vi "SERIAL_StoreBuffer.vi"(8 "error in (no error)":errorcluster, 9 "Access Type":enum16{"set", "get", "delete"}(ring), 10 "navX Data":u8[](array[numeric]), 11 "SerialPortRef":T1) -> (0 "error out":errorcluster, 2 "navX Data":u8[](array[numeric]), 3 "SerialPortRef":T1)   [LabVIEW 2014, in "navX-MXP IMU.lvlib"]
uses:
  navX-MXP IMU.lvlib
  <vilib>/Rock Robotics/WPI/SerialPort/WPI_SerialPortRef.ctl
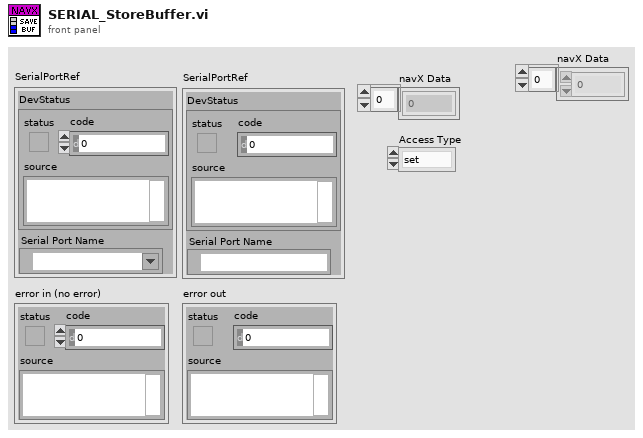
[diagram p1: front panel]
types:
  T1 = typedef "WPI_SerialPortRef.ctl" = cluster{"DevStatus":errorcluster, "Serial Port Name":refnum<visa-resource-name>}
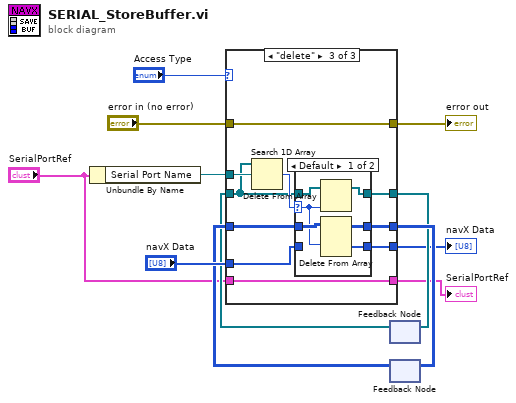
[diagram p0: block diagram]
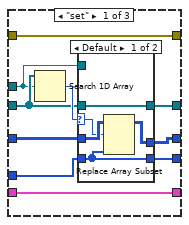
[diagram p2: hidden frame]
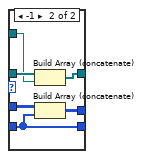
[diagram p3: hidden frame]
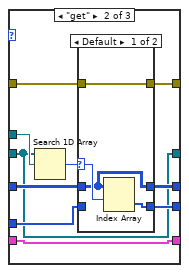
[diagram p4: hidden frame]
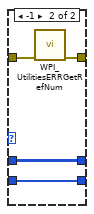
[diagram p5: hidden frame]
diagram:
  n1 = Unbundle By Name("SerialPortRef") -> ("Serial Port Name"=w8:refnum<visa-resource-name>)
  n2 = feedback #1() -> (w7:refnum<visa-resource-name>[])  [unwired: 1 in]
  n3 = feedback #2() -> (w9:u8[][])  [unwired: 1 in]
  n4 = case shown="\"delete\"" "Access Type" {
    tunnel: "navX Data" -> [w21 w36 w53]
    tunnel: [w20 w39 w55] -> w10
    tunnel: w9 -> [w19 w38 w54]
    tunnel: w8 -> [w15 w43 w61]
    tunnel: w7 -> [w17 w35 w58]
    tunnel: [w18 w35 w59] -> w6
    tunnel: [w13 w34 w57] -> w5
    tunnel: "SerialPortRef" -> [w13 w34 w57]
    tunnel: [w16 w40 w56] -> w3
    tunnel: "error in (no error)" -> [w16 w41 w56]
    tunnel: [w14 w37 w52] -> w1
    frame "set" {
      n5 = Search 1D Array(1D array=w17, element=w15) -> (index of element=w22:i32)  [unwired: 1 in]
      n6 = case shown="Default" w22 {
        selector: w22 -> [w23 _]
        tunnel: w21 -> [w24 w28]
        tunnel: [w27 w29] -> w20
        tunnel: w19 -> [w26 w30]
        tunnel: [w25 w31] -> w18
        tunnel: w17 -> [w25 w33]
        tunnel: w15 -> [_ w32]
        tunnel: [w24 w28] -> w14
        frame Default {
          n7 = Replace Array Subset(array=w26, new element=w24, index (row)=w23) -> (w27:u8[][])  [unwired: 1 in]
        }
        frame -1 {
          n8 = Build Array (concatenate)(w33, w32) -> (w31:refnum<visa-resource-name>[])
          n9 = Build Array (concatenate)(w30, w28) -> (w29:u8[][])
        }
      }
    }
    frame "get" {
      n10 = Search 1D Array(1D array=w35, element=w43) -> (index of element=w42:i32)  [unwired: 1 in]
      n11 = case shown="Default" w42 {
        selector: w42 -> [w47 _]
        tunnel: w41 -> [w45 w51]
        tunnel: [w45 w50] -> w40
        tunnel: [w44 w49] -> w39
        tunnel: w38 -> [w44 w49]
        tunnel: [w46 w48] -> w37
        tunnel: w36 -> [_ w48]
        frame Default {
          n12 = Index Array(array=w44, index (row)=w47) -> (element=w46:u8[])  [unwired: 1 in]
        }
        frame -1 {
          n13 = call <vilib>:"WPI_UtilitiesERRGetRefNum.vi"("error in (no error)"=w51) -> ("ERRGetRefNum"=w50:errorcluster)  [unwired: 10 out]
        }
      }
    }
    frame "delete" {
      n14 = Search 1D Array(1D array=w58, element=w61) -> (index of element=w60:i32)  [unwired: 1 in]
      n15 = case shown="Default" w60 {
        selector: w60 -> [w65 _]
        tunnel: [w62 w70] -> w59
        tunnel: w58 -> [w67 w70]
        tunnel: [w64 w69] -> w55
        tunnel: w54 -> [w66 w69]
        tunnel: w53 -> [_ w68]
        tunnel: [w63 w68] -> w52
        frame Default {
          n16 = Delete From Array(array=w67, index=w65) -> (array with subset deleted=w62:refnum<visa-resource-name>[])  [unwired: 1 in, 1 out]
          n17 = Delete From Array(array=w66, index (row)=w65) -> (deleted portion=w63:u8[], array with subset deleted=w64:u8[][])  [unwired: 2 in]
        }
        frame -1 {
        }
      }
    }
  }
  "navX Data" <- w1
  "error out" <- w3
  "SerialPortRef" <- w5
  n18 = feedback-in #1(w6) -> ()
  n19 = feedback-in #2(w10) -> ()
